vi "Parse Response (JSON).vi"(8 "error in":errorcluster, 10 "Response String In":string) -> (0 "error out":errorcluster, 1 "LabVIEW Error?":bool=TRUE, 2 "JSON out":refnum<class "JSON Null.lvclass">)   [LabVIEW 2016, in "JSONRPC Server.lvclass"]
uses:
  JSONRPC Server.lvclass
  <vilib>/NI/JSON Support for LabVIEW/JSON Data Classes/JSON Datatype/JSON Null.lvclass
  <vilib>/NI/JSON Support for LabVIEW/JSON Data Classes/JSON Object/JSON Object.lvclass
  C:/Program Files (x86)/National Instruments/LabVIEW 2016/vi.lib/NI/JSON Support for LabVIEW/JSON Data Classes/JSON Datatype/JSON Null.lvclass
  <vilib>/NI/JSON Support for LabVIEW/JSON Data Classes/JSON Helper/Parsing/Parse Value.vi
  <vilib>/NI/JSON Support for LabVIEW/JSON Data Classes/JSON Helper/To More Specific Type (Object).vi
  <vilib>/NI/JSON Support for LabVIEW/JSON Data Classes/JSON Object/Get Value (JSON).vi
  <vilib>/NI/JSON Support for LabVIEW/JSON Data Classes/JSON Object/Get Value (Object).vi
  <vilib>/NI/JSON Support for LabVIEW/JSON Data Classes/JSON Object/Get Value (Numeric Value).vi
  <vilib>/NI/JSON Support for LabVIEW/JSON Data Classes/JSON Object/Get Value (String Value).vi
  <vilib>/NI/JSON Support for LabVIEW/JSON Data Classes/JSON Helper/JSON Helper.lvclass
  C:/Program Files (x86)/National Instruments/LabVIEW 2016/vi.lib/NI/JSON Support for LabVIEW/JSON Data Classes/JSON Structured Type/JSON Structure.lvclass
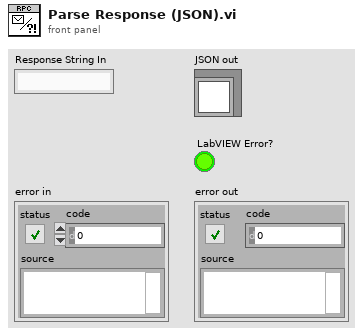
[diagram p1: front panel]
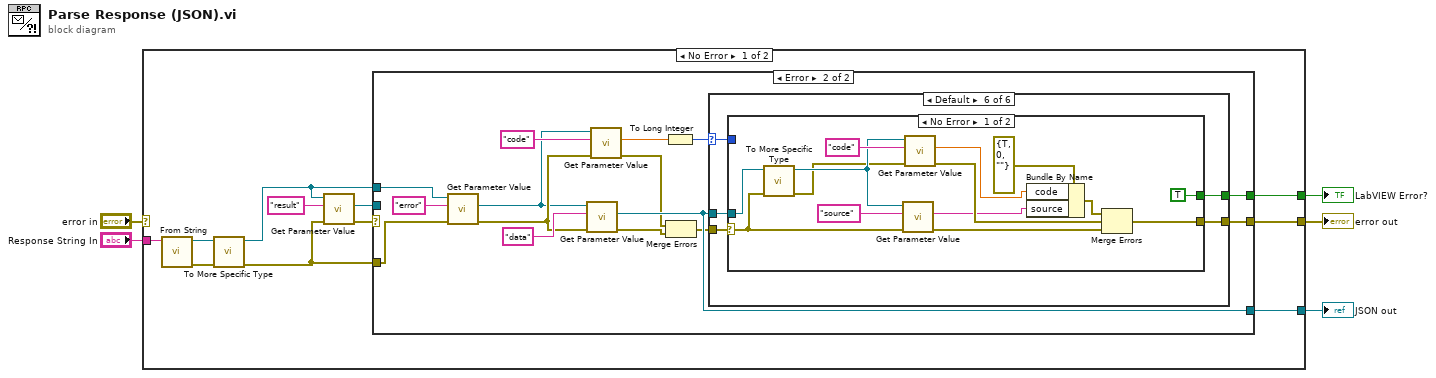
[diagram p0: block diagram]
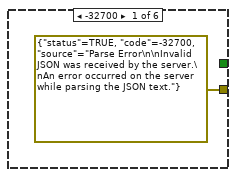
[diagram p3: hidden frame]
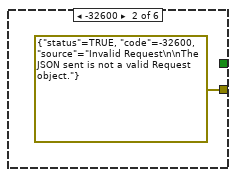
[diagram p4: hidden frame]
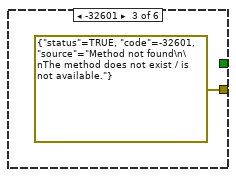
[diagram p5: hidden frame]
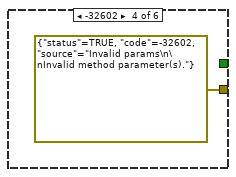
[diagram p6: hidden frame]
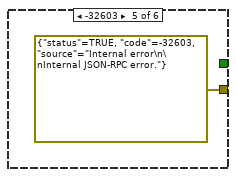
[diagram p7: hidden frame]
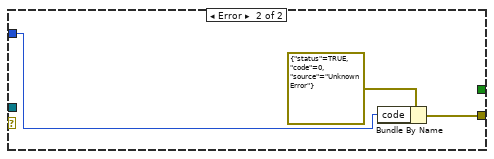
[diagram p8: hidden frame]
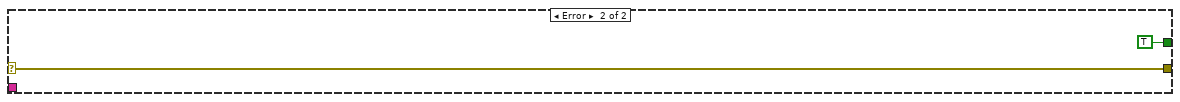
[diagram p9: hidden frame]
diagram:
  n1 = case shown="No Error" "error in" {
    selector: "error in" -> [_ w61]
    tunnel: "Response String In" -> [w13 _]
    tunnel: [w16 _] -> w1
    tunnel: [w15 w61] -> w3
    tunnel: [w14 TRUE] -> w2
    frame No Error {
      n2 = call <vilib>:"From String.vi"("JSON String"=w13) -> ("error out"=w12:errorcluster, "JSON out"=w11:refnum<class "JSON Null.lvclass">)  [unwired: 9 in]
      n3 = call-poly <vilib>:"To More Specific Type.vi"("error in (no error)"=w12, "JSON Datatype in"=w11) -> ("error out"=w6:errorcluster, "JSON Datatype out"=w9:refnum<class "JSON Object.lvclass">)  [unwired: 8 in]
      n4 = call-poly <vilib>:"Get Parameter Value.vi"("error in (no error)"=w6, "key"="result", "JSON Object in"=w9) -> ("error out"=w7:errorcluster, "value"=w8:refnum<class "JSON Null.lvclass">)  [unwired: 7 in]
      n5 = case shown="Error" w7 {
        selector: w7 -> [w17 _]
        tunnel: [w18 w26] -> w16
        tunnel: [w17 w32] -> w15
        tunnel: [_ w31] -> w14
        tunnel: w9 -> [_ w30]
        tunnel: w8 -> [w18 _]
        tunnel: w6 -> [_ w19]
        frame No Error {
        }
        frame Error {
          n6 = call-poly <vilib>:"Get Parameter Value.vi"("error in (no error)"=w19, "key"="error", "JSON Object in"=w30) -> ("error out"=w24:errorcluster, "value"=w21:refnum<class "JSON Object.lvclass">)  [unwired: 7 in]
          n7 = call-poly <vilib>:"Get Parameter Value.vi"("error in (no error)"=w24, "key"="data", "JSON Object in"=w21) -> ("error out"=w23:errorcluster, "value"=w26:refnum<class "JSON Object.lvclass">)  [unwired: 7 in]
          n8 = call-poly <vilib>:"Get Parameter Value.vi"("error in (no error)"=w24, "key"="code", "JSON Object in"=w21) -> ("error out"=w25:errorcluster, "value"=w20:dbl)  [unwired: 7 in]
          n9 = To Long Integer(number=w20) -> (32bit integer=w33:i32)
          n10 = Merge Errors(w25, w23) -> (w22:errorcluster)
          n11 = case shown="Default" w33 {
            selector: w33 -> [_ _ _ _ _ w41]
            tunnel: [errorcluster {"status"=TRUE, "code"=-32700, "source"="Parse Error\n\nInvalid JSON was received by the server.\nAn error occurred on the server while parsing the JSON text."} ("error constant") errorcluster {"status"=TRUE, "code"=-32600, "source"="Invalid Request\n\nThe JSON sent is not a valid Request object."} ("error constant") errorcluster {"status"=TRUE, "code"=-32601, "source"="Method not found\n\nThe method does not exist / is not available."} ("error constant") errorcluster {"status"=TRUE, "code"=-32602, "source"="Invalid params\n\nInvalid method parameter(s)."} ("error constant") errorcluster {"status"=TRUE, "code"=-32603, "source"="Internal error\n\nInternal JSON-RPC error."} ("error constant") w43] -> w32
            tunnel: w26 -> [_ _ _ _ _ w42]
            tunnel: [_ _ _ _ _ w40] -> w31
            tunnel: w22 -> [_ _ _ _ _ w39]
            frame -32700 {
            }
            frame -32600 {
            }
            frame -32601 {
            }
            frame -32602 {
            }
            frame -32603 {
            }
            frame Default {
              n12 = case shown="No Error" w39 {
                selector: w39 -> [w49 _]
                tunnel: [w47 w58] -> w43
                tunnel: w42 -> [w55 _]
                tunnel: w41 -> [_ w59]
                tunnel: [TRUE _] -> w40
                frame No Error {
                  n13 = call-poly <vilib>:"To More Specific Type.vi"("error in (no error)"=w49, "JSON Datatype in"=w55) -> ("error out"=w51:errorcluster, "JSON Datatype out"=w53:refnum<class "JSON Object.lvclass">)  [unwired: 8 in]
                  n14 = call-poly <vilib>:"Get Parameter Value.vi"("error in (no error)"=w49, "key"="source" ("Parameter Name"), "JSON Object in"=w53) -> ("error out"=w50:errorcluster, "value"=w44:string)  [unwired: 7 in]
                  n15 = call-poly <vilib>:"Get Parameter Value.vi"("error in (no error)"=w51, "key"="code", "JSON Object in"=w53) -> ("error out"=w45:errorcluster, "value"=w46:dbl)  [unwired: 7 in]
                  n16 = Bundle By Name(cluster=errorcluster {"status"=TRUE, "code"=0, "source"=""} ("error constant"), "code"=w46, "source"=w44) -> (w48:errorcluster)
                  n17 = Merge Errors(w48, w45, w50) -> (w47:errorcluster)
                }
                frame Error {
                  n18 = Bundle By Name(cluster=errorcluster {"status"=TRUE, "code"=0, "source"="Unknown Error"} ("error constant"), "code"=w59) -> (w58:errorcluster)
                }
              }
            }
          }
        }
      }
    }
    frame Error {
    }
  }
  "error out" <- w3
  "JSON out" <- w1
  "LabVIEW Error?" <- w2
